vi "PCA Normalization.vi"(11 "Original Array":dbl[][](array[numeric])) -> (3 "Zero Mean Array":dbl[][](array[numeric]))   [LabVIEW 2018]
uses:
  <vilib>/Analysis/NI_AALBase.lvlib
panel:
  out "St Dev":dbl[](array[numeric])
  out "Averages":dbl[](array[numeric])
  out "Array Size":i32
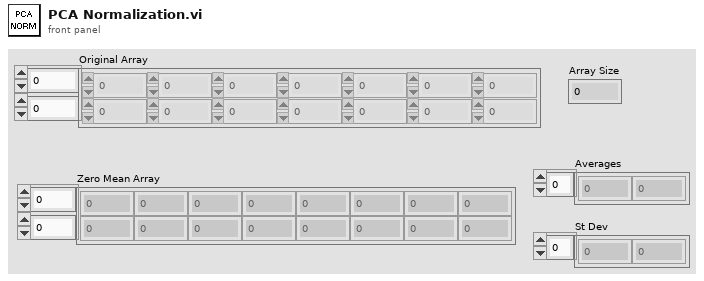
[diagram p1: front panel]
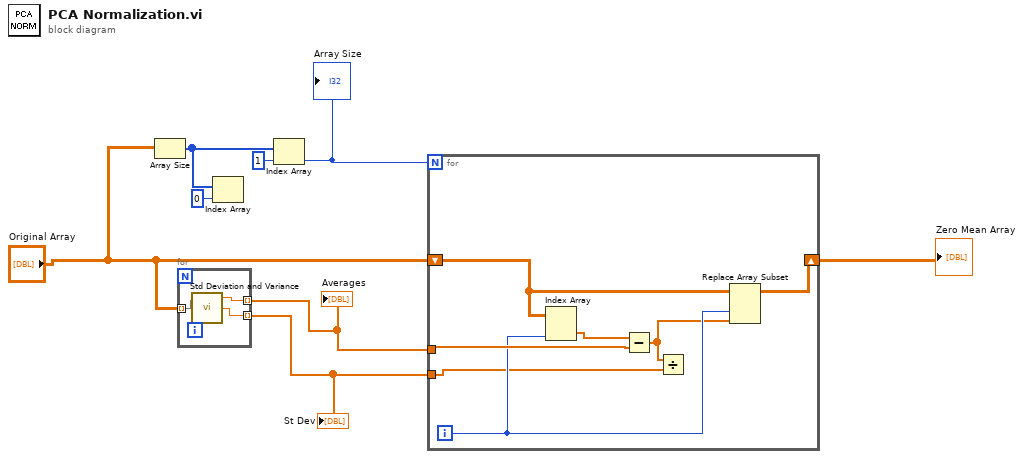
[diagram p0: block diagram]
diagram:
  n1 = Array Size(array="Original Array") -> (size(s)=w6:i32[])
  n2 = for {
    tunnel: "Original Array" -> [w11] mode=indexing
    tunnel: [w10] -> w4 mode=indexing
    tunnel: [w9] -> w2 mode=indexing
    n3 = call <vilib>:"Std Deviation and Variance.vi"("X"=w11) -> ("mean"=w10:dbl, "standard deviation"=w9:dbl)  [unwired: 1 in, 1 out]
  }
  "Averages" <- w4
  "St Dev" <- w2
  n4 = Index Array(array=w6, index=0) -> ()  [unwired: 1 out]
  n5 = Index Array(array=w6, index=1) -> (element=w5:i32)
  "Array Size" <- w5
  n6 = for {
    N: w5 -> [_]
    shift-right: [w15] -> w3
    shift-left: "Original Array" -> [w16]
    tunnel: w4 -> [w17]
    tunnel: w2 -> [w13]
    i -> [w14]
    n7 = Index Array(array=w16, index (col)=w14) -> (element=w18:dbl[])  [unwired: 1 in]
    n8 = Subtract(x=w18, y=w17) -> (x-y=w12:dbl[])
    n9 = Divide(x=w12, y=w13) -> ()  [unwired: 1 out]
    n10 = Replace Array Subset(array=w16, new element=w12, index (col)=w14) -> (w15:dbl[][])  [unwired: 1 in]
  }
  "Zero Mean Array" <- w3
